vi "ColorExceeded.vi"(6 "Init":bool, 8 "error in":errorcluster, 9 "PropGraph":T1={"Raw Data"=[[0.0], [0.0234375], [0.9609375]], "Poperties"={"RMS values"=[], "Max"=[], "Min"=[], "A(8)"=[], "t"=0.0, "A(8) Axis"=0.0, "Aw"=[], "Ak 30min"=0.0, "Ak_axis"=0, "Spec"=[]}, "Power Spectrum / PSD"=[]}, 10 "References":T4, 11 "Value":T3) -> (0 "error out":errorcluster)   [LabVIEW 2019]
uses:
  TypeDef/#TypeDef_References.ctl
  TypeDef/#TypeDef_Buttons.ctl
  TypeDef/#TypeDef_ReferencesMeassurementProp.ctl
  TypeDef/#TypeDef_ReferencesArchiveProp.ctl
  TypeDef/#TypeDef_Lists.ctl
  TypeDef/#TypeDef_MeasProp.ctl
  TypeDef/#TypeDef_OpProp.ctl
  TypeDef/#TypeDef_Enum_ModeOp.ctl
  TypeDef/#TypeDef_Enum_Buttons.ctl
  Communication/TypeDef/#TypeDef_PropGraph.ctl
  Communication/TypeDef/#TypeDef_PropertiesToSave.ctl
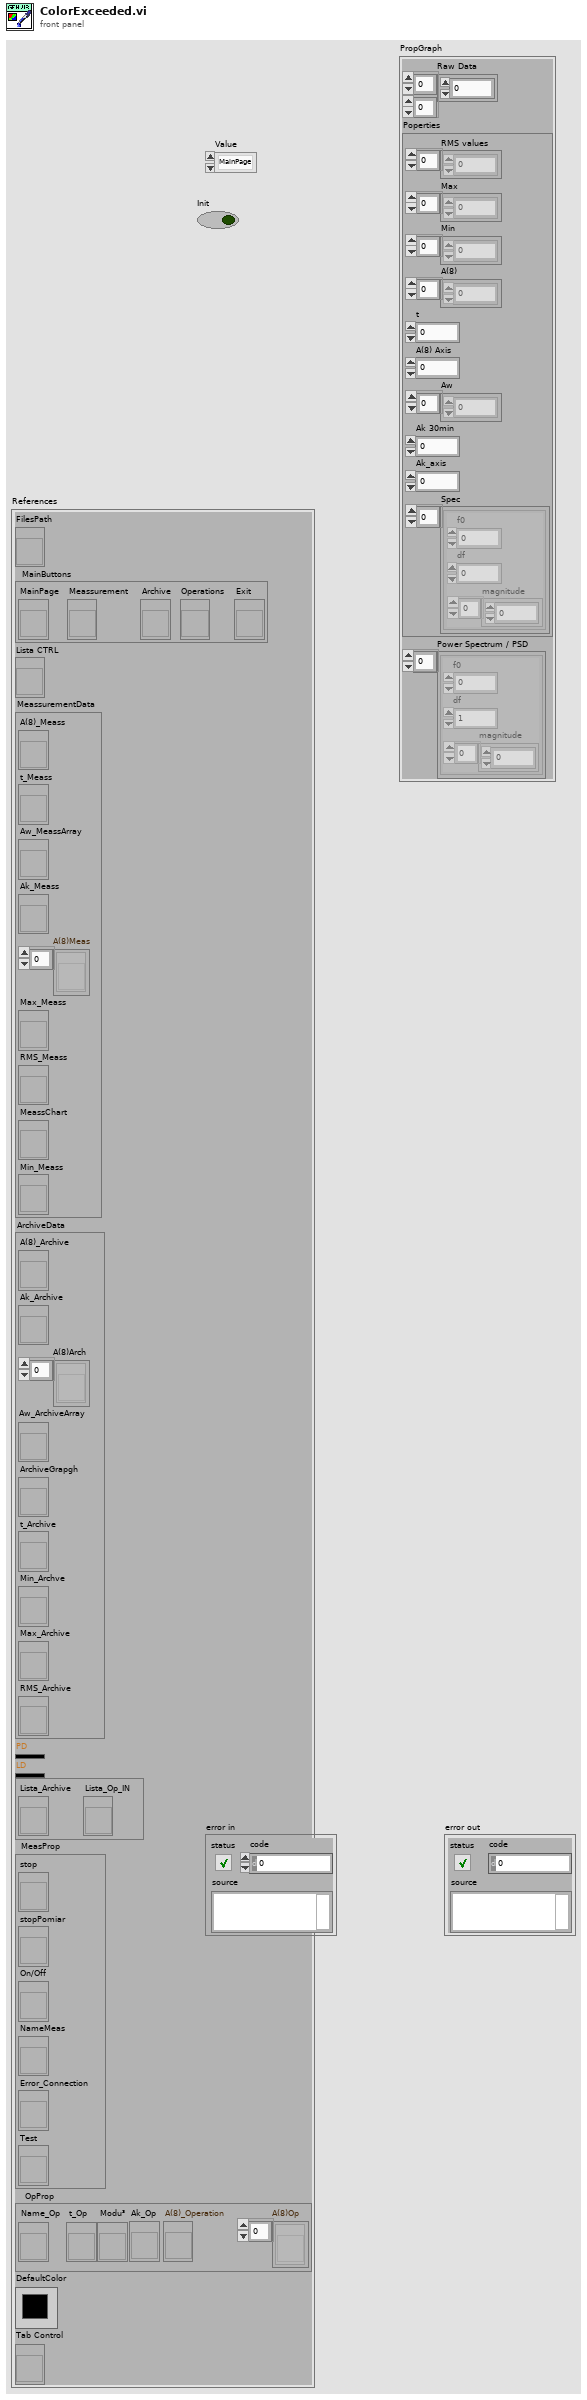
[diagram p1: front panel]
types:
  T1 = typedef "#TypeDef_PropGraph.ctl" = cluster{"Raw Data":dbl[][], "Poperties":T2, "Power Spectrum / PSD":cluster{"f0":dbl, "df":dbl, "magnitude":dbl[]}[]}
  T2 = typedef "#TypeDef_PropertiesToSave.ctl" = cluster{"RMS values":dbl[], "Max":dbl[], "Min":dbl[], "A(8)":dbl[], "t":dbl, "A(8) Axis":dbl, "Aw":dbl[], "Ak 30min":dbl, "Ak_axis":i32, "Spec":cluster{"f0":dbl, "df":dbl, "magnitude":dbl[]}[]}
  T3 = typedef "#TypeDef_Enum_Buttons.ctl" = enum32{"MainPage", "Pomiar", "Archiwum", "Operacje", "Wyjœcie"}
  T4 = typedef "#TypeDef_References.ctl" = cluster{"FilesPath":refnum<vi>, "MainButtons":T5, "Lista CTRL":refnum<vi>, "MeassurementData":T6, "ArchiveData":T7, "PD":u32, "LD":u32, "Lists":T8, "MeasProp":T9, "OpProp":T10, "DefaultColor":u32, "Tab Control":refnum<vi>}
  T5 = typedef "#TypeDef_Buttons.ctl" = cluster{"MainPage":refnum<vi>, "Meassurement":refnum<vi>, "Archive":refnum<vi>, "Operations":refnum<vi>, "Exit":refnum<vi>}
  T6 = typedef "#TypeDef_ReferencesMeassurementProp.ctl" = cluster{"A(8)_Meass":refnum<vi>, "t_Meass":refnum<vi>, "Aw_MeassArray":refnum<vi>, "Ak_Meass":refnum<vi>, "A(8)Meas":refnum<vi>[], "Max_Meass":refnum<vi>, "RMS_Meass":refnum<vi>, "MeassChart":refnum<vi>, "Min_Meass":refnum<vi>}
  T7 = typedef "#TypeDef_ReferencesArchiveProp.ctl" = cluster{"A(8)_Archive":refnum<vi>, "Ak_Archive":refnum<vi>, "A(8)Arch":refnum<vi>[], "Aw_ArchiveArray":refnum<vi>, "ArchiveGrapgh":refnum<vi>, "t_Archive":refnum<vi>, "Min_Archve":refnum<vi>, "Max_Archive":refnum<vi>, "RMS_Archive":refnum<vi>}
  T8 = typedef "#TypeDef_Lists.ctl" = cluster{"Lista_Archive":refnum<vi>, "Lista_Op_IN":refnum<vi>}
  T9 = typedef "#TypeDef_MeasProp.ctl" = cluster{"stop":refnum<vi>, "stopPomiar":refnum<vi>, "On/Off":refnum<vi>, "NameMeas":refnum<vi>, "Error_Connection":refnum<vi>, "Test":refnum<vi>}
  T10 = typedef "#TypeDef_OpProp.ctl" = cluster{"Name_Op":refnum<vi>, "t_Op":refnum<vi>, "Modu³":refnum<vi>, "Ak_Op":refnum<vi>, "A(8)_Operation":refnum<vi>, "A(8)Op":refnum<vi>[]}
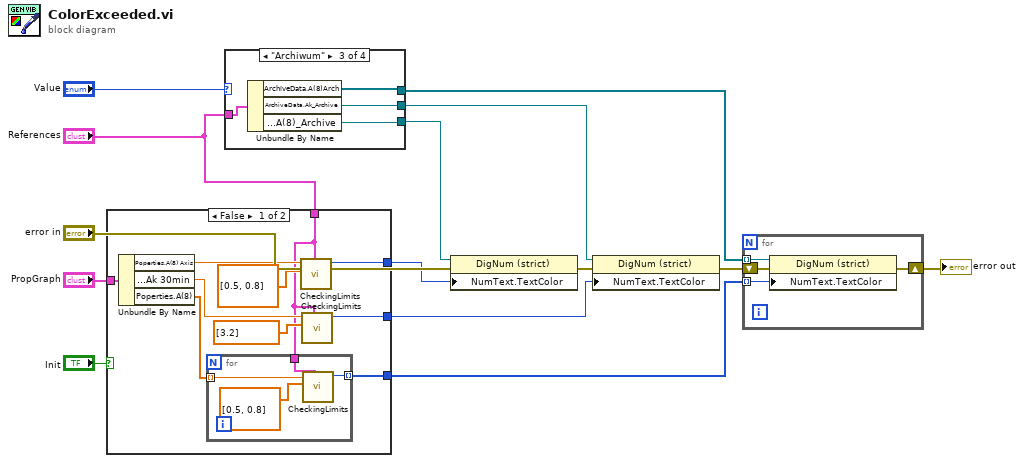
[diagram p0: block diagram]
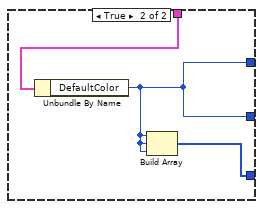
[diagram p2: hidden frame]
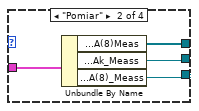
[diagram p4: hidden frame]
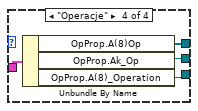
[diagram p5: hidden frame]
diagram:
  n1 = case shown="False" "Init" {
    tunnel: [w24 w29] -> w13
    tunnel: [w19 w29] -> w8
    tunnel: "PropGraph" -> [w18 _]
    tunnel: "References" -> [w17 w31]
    tunnel: [w15 w30] -> w2
    frame False {
      n2 = Unbundle By Name(w18) -> ("Poperties.A(8) Axis"=w22:dbl, "Poperties.Ak 30min"=w21:dbl, "Poperties.A(8)"=w16:dbl[])
      n3 = for {
        tunnel: w17 -> [w27]
        tunnel: w16 -> [w26] mode=indexing
        tunnel: [w25] -> w15 mode=indexing
        n4 = call "CheckingLimits.vi"("References"=w27, "Limits"=dbl[] [0.5, 0.8], "Data"=w26) -> ("Color"=w25:u32)  [unwired: 8 in]
      }
      n5 = call "CheckingLimits.vi"("References"=w17, "Limits"=dbl[] [0.5, 0.8], "Data"=w22) -> ("Color"=w24:u32)  [unwired: 8 in]
      n6 = call "CheckingLimits.vi"("References"=w17, "Limits"=dbl[] [3.2], "Data"=w21) -> ("Color"=w19:u32)  [unwired: 8 in]
    }
    frame True {
      n7 = Unbundle By Name(w31) -> ("DefaultColor"=w29:u32)
      n8 = Build Array(w29, w29, w29) -> (w30:u32[])
    }
  }
  n9 = case shown="\"Archiwum\"" "Value" {
    tunnel: "References" -> [_ w35 w39 w43]
    tunnel: [_ w34 w38 w41] -> w12
    tunnel: [_ w33 w37 w42] -> w9
    tunnel: [_ w32 w36 w40] -> w5
    frame "MainPage", Default {
    }
    frame "Pomiar" {
      n10 = Unbundle By Name(w35) -> ("MeassurementData.A(8)Meas"=w32:refnum<vi>[], "MeassurementData.Ak_Meass"=w33:refnum<vi>, "MeassurementData.A(8)_Meass"=w34:refnum<vi>)
    }
    frame "Archiwum" {
      n11 = Unbundle By Name(w39) -> ("ArchiveData.A(8)Arch"=w36:refnum<vi>[], "ArchiveData.Ak_Archive"=w37:refnum<vi>, "ArchiveData.A(8)_Archive"=w38:refnum<vi>)
    }
    frame "Operacje" {
      n12 = Unbundle By Name(w43) -> ("OpProp.A(8)Op"=w40:refnum<vi>[], "OpProp.Ak_Op"=w42:refnum<vi>, "OpProp.A(8)_Operation"=w41:refnum<vi>)
    }
  }
  n13 = property class="DigNum (strict)"(reference=w12, error in="error in", "NumText.TextColor"=w13) -> (error out=w10:errorcluster)  [unwired: 1 out]
  n14 = property class="DigNum (strict)"(reference=w9, error in=w10, "NumText.TextColor"=w8) -> (error out=w6:errorcluster)  [unwired: 1 out]
  n15 = for {
    tunnel: w5 -> [w46] mode=indexing
    shift-right: [w45] -> w4
    shift-left: w6 -> [w47]
    tunnel: w2 -> [w44] mode=indexing
    n16 = property class="DigNum (strict)"(reference=w46, error in=w47, "NumText.TextColor"=w44) -> (error out=w45:errorcluster)  [unwired: 1 out]
  }
  "error out" <- w4
